vi "Run.vi"(7 "Team Index":i32, 8 "Column":i32, 9 "Row":i32, 10 "View":i32[](array[numeric]) caption="View (Team Index, -1: empty)", 11 "Starter In":refnum<class "Starter.lvclass">) -> (0 "Replicated":refnum<class "Square.lvclass">, 1 "Direction":T1, 2 "Action":T2, 3 "Square Out":refnum<class "Square.lvclass">)   [LabVIEW 2015, in "Starter.lvclass"]
uses:
  Starter.lvclass
  Square/Square.lvclass
  Type Defs/Action Enum.ctl
  Type Defs/Direction Enum.ctl
  Common/Position.ctl
  Wall/Permanent Wall.lvclass
  Type Defs/SB Type Defs.lvlib
  Fortress/Fortress.lvclass
  Common/Common.lvlib
panel:
  # "NW\nN\nNE\nE\nSE\nS\nSW\nW"
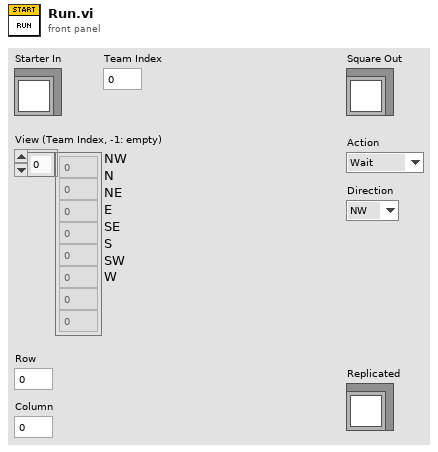
[diagram p1: front panel]
types:
  T1 = typedef "SB Type Defs.lvlib/Direction Enum.ctl" = enum16{"NW", "N", "NE", "E", "SE", "S", "SW", "W"}
  T2 = typedef "SB Type Defs.lvlib/Action Enum.ctl" = enum16{"Wait", "Move", "Attack", "Replicate"}
  T3 = typedef "Common.lvlib/Position.ctl" = cluster{"Column":i32, "Row":i32}
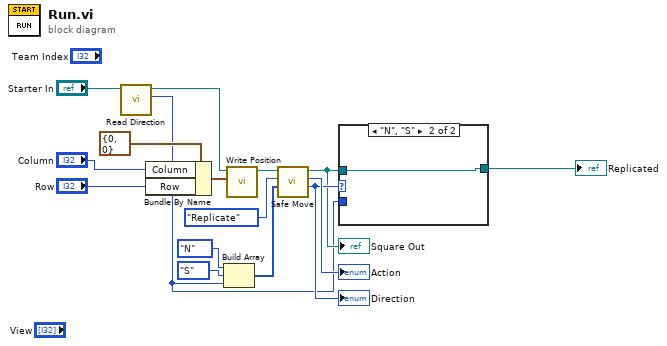
[diagram p0: block diagram]
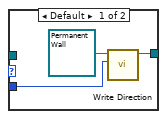
[diagram p2: hidden frame]
diagram:
  n1 = call-dynamic "Read Direction.vi"("Fortress in"="Starter In") -> ("Direction"=w1:T1, "Fortress out"=w2:refnum<class "Starter.lvclass">)  [unwired: 8 in, 1 out]
  n2 = Bundle By Name(cluster=T3 {"Column"=0, "Row"=0} ("Position"), "Column"="Column", "Row"="Row") -> (w4:T3)
  n3 = Build Array(Direction_Enum."N" ("Direction"), Direction_Enum."S" ("element"), w1) -> (w14:T1[])
  n4 = call-dynamic "Write Position.vi"("Position"=w4, "Fortress in"=w2) -> ("Fortress out"=w6:refnum<class "Starter.lvclass">)  [unwired: 8 in, 1 out]
  n5 = call "Safe Move.vi"("Directions in"=w14, "Action in"=Action_Enum."Replicate", "Fortress In"=w6) -> ("Direction"=w11:T1, "Action out"=→"Action":T2, "Fortress Out"=w9:refnum<class "Starter.lvclass">)  [unwired: 5 in, 1 out]
  "Square Out" <- w9
  "Direction" <- w11
  n6 = case shown="\"N\", \"S\"" w11 {
    tunnel: [w18 w20] -> w10
    tunnel: w9 -> [_ w20]
    tunnel: w1 -> [w17 _]
    frame Default {
      n7 = call-dynamic "Write Direction.vi"("Direction"=w17, "Permanent Wall in"=refnum<class "Permanent Wall.lvclass"> refnum ("Permanent Wall.lvclass")) -> ("Permanent Wall out"=w18:refnum<class "Permanent Wall.lvclass">)  [unwired: 8 in, 1 out]
    }
    frame "N", "S" {
    }
  }
  "Replicated" <- w10
